vi "read.vi"(6 "timeout (0)":i32, 8 "error in (no error)":errorcluster, 9 "bufferSize":i64, 10 "signalCount":i32, 11 "IMultiReader in":refnum<class "IMultiReader.lvclass">) -> (0 "error out":errorcluster, 1 "Multi Reader Status out":refnum<class "IMultiReaderStatus.lvclass">, 2 "Read Buffers out":dbl[][](array[numeric]), 3 "IMultiReader out":refnum<class "IMultiReader.lvclass">)   [LabVIEW 2022 SP3, in "openDAQ.lvlib" / "IBaseObject.lvlib" / "IReader.lvlib" / "ISampleReader.lvlib" / "IMultiReader.lvlib" / "IMultiReader.lvclass"]
uses:
  <instrlib>/openDAQ/Public/Classes/IMultiReader/IMultiReader.lvclass
  C:/Program Files (x86)/National Instruments/LabVIEW 2022/instr.lib/openDAQ/Public/Classes/IBaseObject/IBaseObject.lvclass
  <instrlib>/openDAQ/Public/Classes/IMultiReaderStatus/IMultiReaderStatus.lvclass
  <instrlib>/openDAQ/Public/Classes/IBaseObject/IBaseObject.lvclass/IBaseObject.ctl
  <instrlib>/openDAQ/Public/Classes/IBaseObject/Accessor/Read reference.vi
  <instrlib>/openDAQ/Public/Classes/IBaseObject/Accessor/Write reference.vi
  <instrlib>/openDAQ/Binaries/Windows/x86/copendaq32.dll
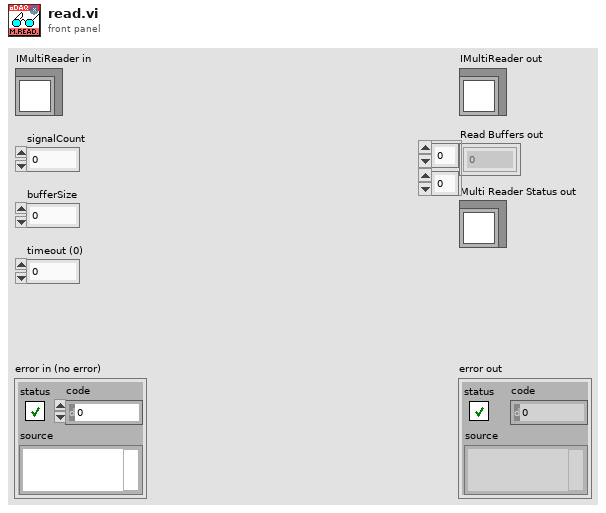
[diagram p1: front panel]
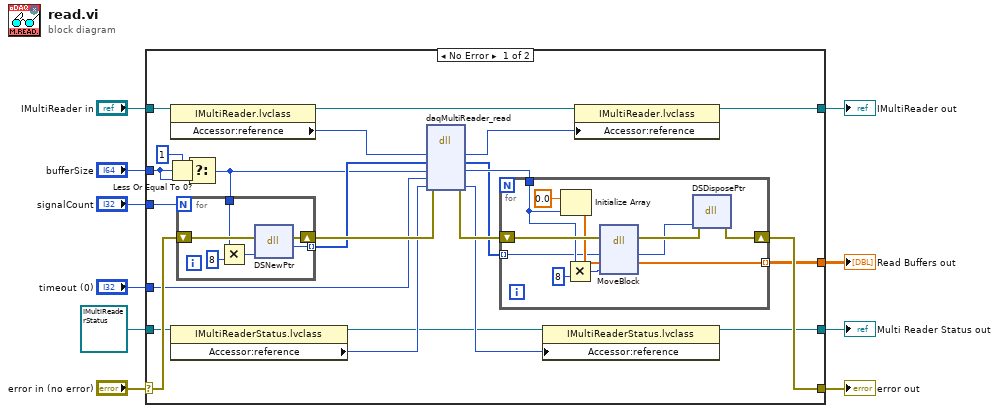
[diagram p0: block diagram]
diagram:
  n1 = case shown="No Error" "error in (no error)" {
    selector: "error in (no error)" -> [w31 w54]
    tunnel: [w34 w54] -> w9
    tunnel: [w28 w53] -> w7
    tunnel: "IMultiReader in" -> [w30 w53]
    tunnel: "bufferSize" -> [w15 _]
    tunnel: refnum<class "IMultiReaderStatus.lvclass"> refnum ("openDAQ.lvlib:IBaseObject.lvlib:IReaderStatus.lvlib:IMultiReaderStatus.lvlib:IMultiReaderStatus.lvclass") -> [w25 w52]
    tunnel: [w21 w52] -> w4
    tunnel: "timeout (0)" -> [w20 _]
    tunnel: "signalCount" -> [w19 _]
    tunnel: [w11 _] -> w1
    frame No Error {
      n2 = Less Or Equal To 0?(x=w15) -> (x <= 0?=w17:bool)
      n3 = property class="IMultiReader.lvclass"(reference=w30) -> (reference out=w29:refnum<class "IMultiReader.lvclass">, "Accessor:reference"=w27:i64)  [unwired: 1 in, 1 out]
      n4 = property class="IMultiReaderStatus.lvclass"(reference=w25) -> (reference out=w22:refnum<class "IMultiReaderStatus.lvclass">, "Accessor:reference"=w24:i64)  [unwired: 1 in, 1 out]
      n5 = Select(t=i64 1, s=w17, f=w15) -> (s? t:f=w16:i64)
      n6 = for {
        N: w19 -> [_]
        tunnel: w16 -> [w48]
        shift-right: [w50] -> w32
        shift-left: w31 -> [w51]
        tunnel: [w46] -> w18 mode=indexing
        n7 = Multiply(x=w48, y=i64 8) -> (x*y=w47:i64)
        n8 = dll-call lib="LabVIEW" fn="DSNewPtr"(error in=w51, "size"=w47) -> (error out=w50:errorcluster, "block*"=w46:i64)  [unwired: 3 in, 1 out]
      }
      n9 = dll-call lib="C:/Program Files (x86)/National Instruments/LabVIEW 2022/instr.lib/openDAQ/Binaries/Windows/x86/copendaq*.*" fn="daqMultiReader_read"(error in=w32, "multiReader"=w27, "dataBuffers"=w18, "count"=w16, "timeout"=w20, "status"=w24) -> (error out=w33:errorcluster, "multiReader"=w26:i64, "dataBuffers"=w12:i64[], "count"=w13:i64, "status"=w23:i64)  [unwired: 4 in, 1 out]
      n10 = for {
        tunnel: w13 -> [w41]
        shift-right: [w37] -> w34
        shift-left: w33 -> [w44]
        tunnel: w12 -> [w39] mode=indexing
        tunnel: [w35] -> w11 mode=indexing
        n11 = Initialize Array(0.0 ("element"), w41) -> (w40:dbl[])
        n12 = Multiply(x=w41, y=i64 8) -> (x*y=w43:i64)
        n13 = dll-call lib="LabVIEW" fn="MoveBlock"(error in=w44, "start"=w39, "destination"=w40, "size"=w43) -> (error out=w38:errorcluster, "start"=w36:i64, "destination"=w35:dbl[])  [unwired: 4 in, 1 out]
        n14 = dll-call lib="LabVIEW" fn="DSDisposePtr"(error in=w38, "pointer"=w36) -> (error out=w37:errorcluster)  [unwired: 4 in, 1 out]
      }
      n15 = property class="IMultiReaderStatus.lvclass"(reference=w22, "Accessor:reference"=w23) -> (reference out=w21:refnum<class "IMultiReaderStatus.lvclass">)  [unwired: 1 in, 1 out]
      n16 = property class="IMultiReader.lvclass"(reference=w29, "Accessor:reference"=w26) -> (reference out=w28:refnum<class "IMultiReader.lvclass">)  [unwired: 1 in, 1 out]
    }
    frame Error {
    }
  }
  "error out" <- w9
  "IMultiReader out" <- w7
  "Multi Reader Status out" <- w4
  "Read Buffers out" <- w1
